vi "pre-set-conditional-disable.vi"(6 "Top Level/Always Included VIs":path[](array[path]), 7 "Main Destination Path":path, 9 "Target Name":string, 10 "Build Specification Name":string, 11 "Project Path":path) -> (0 "error out":errorcluster)   [LabVIEW 2019]
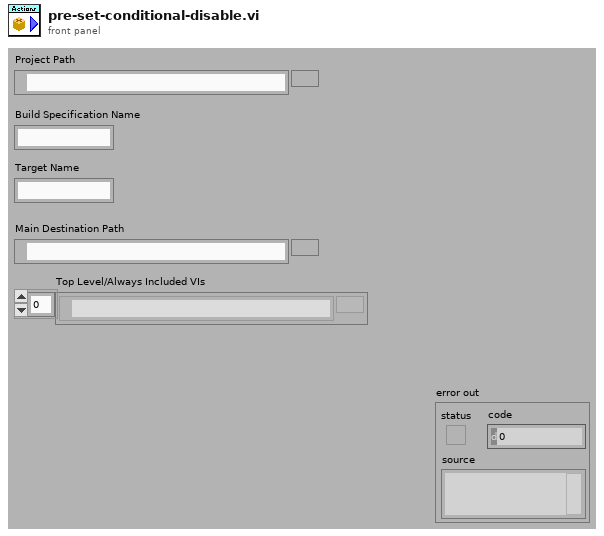
[diagram p1: front panel]
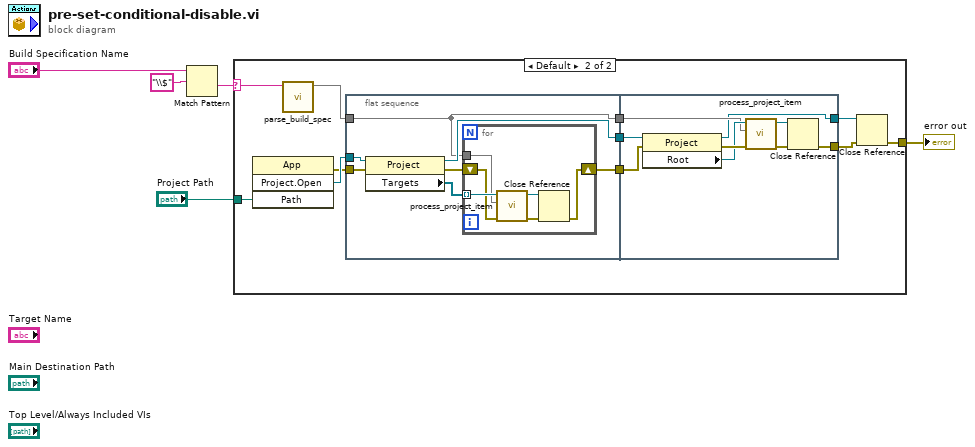
[diagram p0: block diagram]
diagram:
  n1 = Match Pattern(string="Build Specification Name", regular expression="\\$") -> (after substring=w1:string)  [unwired: 1 in, 3 out]
  n2 = case shown="Default" w1 {
    selector: w1 -> [_ w14]
    tunnel: "Project Path" -> [_ w15]
    tunnel: [_ w16] -> w2
    frame "" {
    }
    frame Default {
      n3 = invoke class="App" method="Project.Open"("Path"=w15) -> (error out=w6:errorcluster, "Project:Open"=w7:refnum<vi>)  [unwired: 3 in, 2 out]
      n4 = call "parse_build_spec.vi"("build spec symbols"=w14) -> ("CCSymbols"=w8:map{string, string})  [unwired: 10 in]
      n5 = flat-sequence {
        tunnel: [w22] -> w11
        tunnel: [w20] -> w10
        tunnel: [w19] -> w9
        tunnel: w8 -> [w19]
        tunnel: w7 -> [w18]
        tunnel: w6 -> [w17]
        tunnel: [w31] -> w12
        tunnel: [w30] -> w13
        tunnel: w11 -> [w34]
        tunnel: w10 -> [w33]
        tunnel: w9 -> [w32]
        frame #0 {
          n6 = property class="Project"(reference=w18, error in=w17) -> (reference out=w22:refnum<vi>, error out=w21:errorcluster, "Targets"=w23:refnum<vi>[])
          n7 = for {
            tunnel: w23 -> [w29] mode=indexing
            tunnel: w19 -> [w28]
            shift-right: [w24] -> w20
            shift-left: w21 -> [w25]
            n8 = call "process_project_item.vi"("error in (no error)"=w25, "CCSymbols"=w28, "ProjectItem in"=w29) -> ("error out"=w26:errorcluster, "ProjectItem out"=w27:refnum<vi>)  [unwired: 7 in]
            n9 = Close Reference(reference=w27, error in (no error)=w26) -> (error out=w24:errorcluster)
          }
        }
        frame #1 {
          n10 = property class="Project"(reference=w34, error in=w33) -> (reference out=w30:refnum<vi>, error out=w38:errorcluster, "Root"=w37:refnum<vi>)
          n11 = call "process_project_item.vi"("error in (no error)"=w38, "CCSymbols"=w32, "ProjectItem in"=w37) -> ("error out"=w36:errorcluster, "ProjectItem out"=w35:refnum<vi>)  [unwired: 7 in]
          n12 = Close Reference(reference=w35, error in (no error)=w36) -> (error out=w31:errorcluster)
        }
      }
      n13 = Close Reference(reference=w13, error in (no error)=w12) -> (error out=w16:errorcluster)
    }
  }
  "error out" <- w2
